vi "Configure Function.vi"(7 "Function":u16(ring) items=["DCI", "DCV"], 8 "error in (no error)":errorcluster, 11 "Keithley 2000 in":refnum<class "Keithley 2000.lvclass">) -> (0 "error out":errorcluster, 3 "Keithley 2000 out":refnum<class "Keithley 2000.lvclass">)   [LabVIEW 2020, in "Keithley 2000.lvclass"]
uses:
  Keithley 2000.lvclass
  C:/Sandbox/RF Bench/Source Code/WiSpry Test Framework/Instruments/Instrument.lvclass
  C:/Sandbox/RF Bench/Source Code/WiSpry Test Framework/Instruments/Digital Multimeter/Digital Multimeter.lvclass
  Instrument.lvclass/Instrument.ctl
  Digital Multimeter.lvclass/Digital Multimeter.ctl
  <instrlib>/Keithley 2000/Public/Configure/Configure DC Volts.vi
  <instrlib>/Keithley 2000/Public/Configure/Configure DC Current.vi
  Instrument.lvclass
  <instrlib>/Keithley 2000/Keithley 2000.lvlib
  Digital Multimeter.lvclass
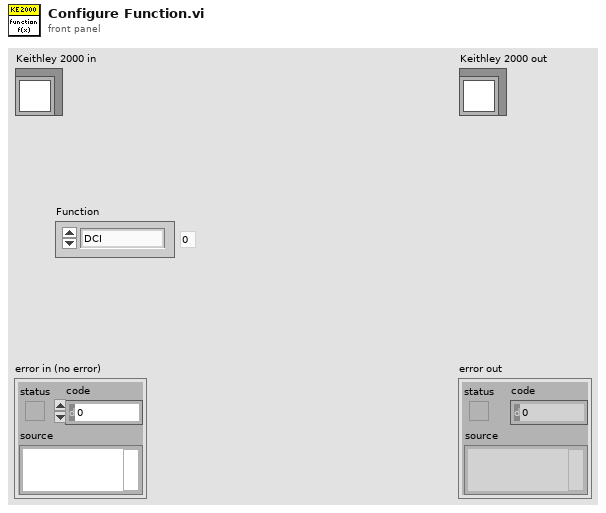
[diagram p1: front panel]
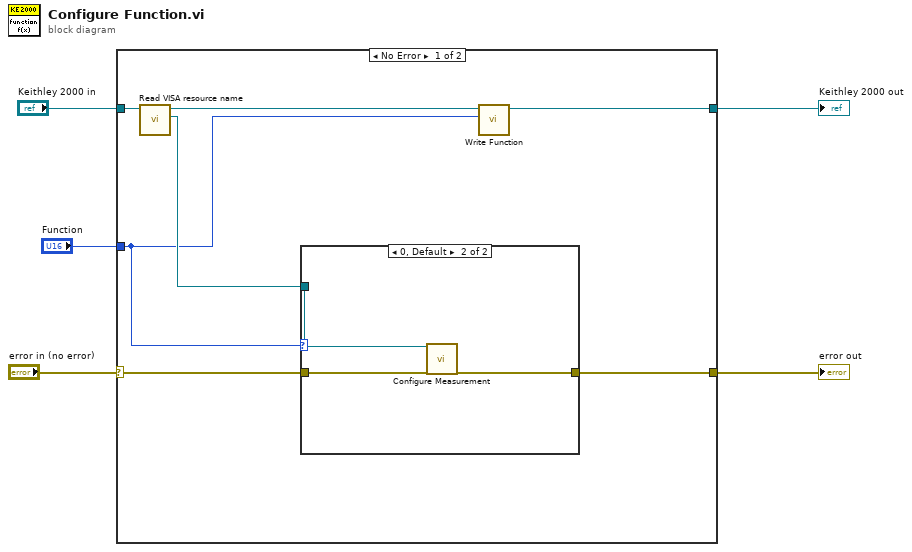
[diagram p0: block diagram]
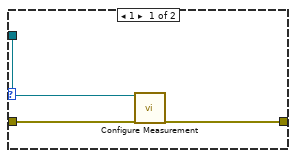
[diagram p2: hidden frame]
diagram:
  n1 = case shown="No Error" "error in (no error)" {
    selector: "error in (no error)" -> [w9 w20]
    tunnel: [w10 w20] -> w4
    tunnel: [w6 w19] -> w3
    tunnel: "Keithley 2000 in" -> [w12 w19]
    tunnel: "Function" -> [w8 _]
    frame No Error {
      n2 = call "Read VISA resource name.vi"("Instrument in"=w12) -> ("VISA resource name"=w11:refnum<visa-resource-name>, "Instrument out"=w7:refnum<class "Keithley 2000.lvclass">)  [unwired: 9 in]
      n3 = case shown="0, Default" w8 {
        tunnel: w11 -> [w15 w18]
        tunnel: [w14 w17] -> w10
        tunnel: w9 -> [w13 w16]
        frame 1 {
          n4 = call-poly <instrlib>:"Configure Measurement.vi"("VISA resource name"=w15, "error in (no error)"=w13) -> ("error out"=w14:errorcluster)  [unwired: 16 in, 1 out]
        }
        frame 0, Default {
          n5 = call-poly <instrlib>:"Configure Measurement.vi"("VISA resource name"=w18, "error in (no error)"=w16) -> ("error out"=w17:errorcluster)  [unwired: 16 in, 1 out]
        }
      }
      n6 = call "Write Function.vi"("Function"=w8, "Digtal Multimeter in"=w7) -> ("Digtal Multimeter out"=w6:refnum<class "Keithley 2000.lvclass">)  [unwired: 9 in]
    }
    frame Error {
    }
  }
  "error out" <- w4
  "Keithley 2000 out" <- w3
